vi "list+Graph with Splitter Bars.vi"() -> ()   [LabVIEW 2013]
doc: "该范例演示了在前面板上使用分隔栏，创建多个窗格的方法。依据窗格的功能，可为窗格设置不同的动作。在本范例中，右下角窗格中的图形控件可调整大小以匹配所属窗格。"
uses:
  <vilib>/measure/NI_MABase.lvlib
panel:
  in  "选择波形":i32(listbox)
  out "显示消息":string
  in  "停止":bool
  in  "清除":bool
  in  "加载":bool
  out "波形图":waveform(dbl)(graph)
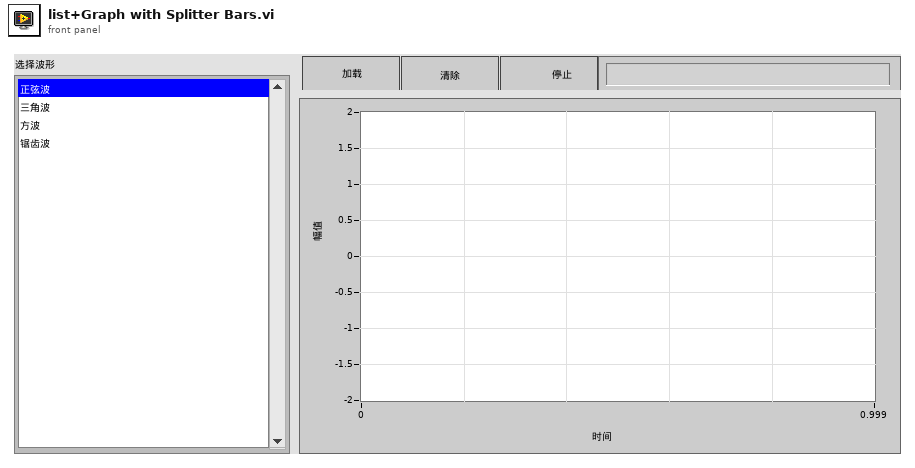
[diagram p1: front panel]
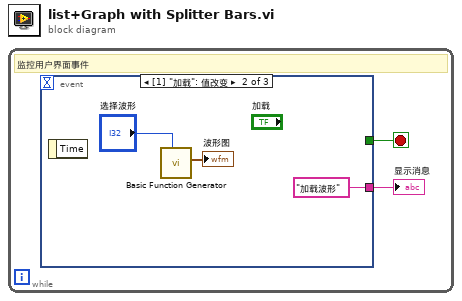
[diagram p0: block diagram]
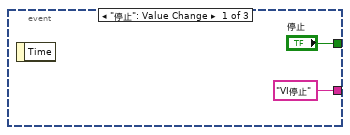
[diagram p2: hidden frame]
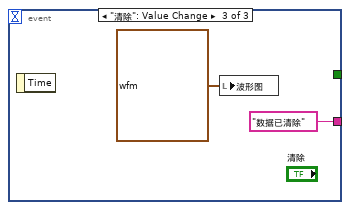
[diagram p3: hidden frame]
diagram:
  n1 = while {
    stop <- w2 stop-if-true
    # "监控用户界面事件"
    n2 = event shown="[1] \"加载\": 值改变" {
      selector: _ -> [_ _ _]
      dyn-events: _ -> [_ _ _]
      timeout: _ -> [_ _ _]
      tunnel: ["停止" _ _] -> w2
      tunnel: ["VI停止" ("停止消息") "加载波形" ("清除消息") "数据已清除" ("清除消息")] -> w1
      event "停止": Value Change {
        n3 = event-data() -> ()  [unwired: 1 in, 1 out]
      }
      event "加载": Value Change {
        n4 = event-data() -> ()  [unwired: 1 in, 1 out]
        n5 = call <vilib>:"Basic Function Generator.vi"("signal type"="选择波形") -> ("signal out"=→"波形图":waveform(dbl))  [unwired: 8 in, 2 out]
      }
      event "清除": Value Change {
        n6 = event-data() -> ()  [unwired: 1 in, 1 out]
        n7 = local write "波形图"(waveform(dbl) {"t0"=timestamp(0 s since 1904-01-01), "dt"=1.0, "Y"=[]} ("波形图")) -> ()
      }
    }
    "显示消息" <- w1
  }
